vi "ESC Run VI Named.vi"(3 "Mode":T5=enum."Run VI", 5 "Traverse line In":T2={"Start X"=0.0, "Start Y"=0.0, "Start Z"=0.0, "End X"=0.0, "End Y"=0.0, "End Z"=0.0, "nPoints"=0, "Spacing"=enum."Linear", "Filename"=path "", "Tunnel Speed"=0.0, "Averaging time (mins)"=0.0, "Extra Commands"="", "Carrier_1 Q (l/min)"=0.0, "Carrier_2 Q (l/min)"=0.0, "Trace Gas Concentration (%)"=0.0, "Specific Arguments"="Source_Live_Control.vi; 1", "Comments"="", "Row No"=0, "Row Type Selector"=enum."Move Traverse Only", "EstCompl"="", "Row Duration (mins)"=0.0, "nValidPoints"=0, "Meas Setup File"=""} {"Carrier_2 Q (l/min)" format="%#.2f"; "Row Duration (mins)" format="%#.1f"; "Row No" min=0; "Trace Gas Concentration (%)" min=0.0 format="%#_4f"; "Carrier_1 Q (l/min)" format="%#.4f"; "Start X" format="%#.2f"; "Start Y" format="%#.2f"; "Start Z" format="%#.2f"; "End X" format="%#.2f"; "End Y" format="%#.2f"; "End Z" format="%#.2f"; "Tunnel Speed" format="%#.2f"; "Averaging time (mins)" min=0.0 format="%#.2f"}) -> (0 "Error Message":string, 1 "Status":T1, 2 "Traverse line Out":T2={"Start X"=0.0, "Start Y"=0.0, "Start Z"=0.0, "End X"=0.0, "End Y"=0.0, "End Z"=0.0, "nPoints"=0, "Spacing"=enum."Linear", "Filename"=path "", "Tunnel Speed"=0.0, "Averaging time (mins)"=0.0, "Extra Commands"="", "Carrier_1 Q (l/min)"=0.0, "Carrier_2 Q (l/min)"=0.0, "Trace Gas Concentration (%)"=0.0, "Specific Arguments"="Source_Live_Control.vi; 1", "Comments"="", "Row No"=0, "Row Type Selector"=enum."Move Traverse Only", "EstCompl"="", "Row Duration (mins)"=0.0, "nValidPoints"=0, "Meas Setup File"=""} {"Carrier_2 Q (l/min)" format="%#.2f"; "Row Duration (mins)" format="%#.1f"; "Row No" min=0; "Trace Gas Concentration (%)" min=0.0 format="%#_4f"; "Carrier_1 Q (l/min)" format="%#.4f"; "Start X" format="%#.2f"; "Start Y" format="%#.2f"; "Start Z" format="%#.2f"; "End X" format="%#.2f"; "End Y" format="%#.2f"; "End Z" format="%#.2f"; "Tunnel Speed" format="%#.2f"; "Averaging time (mins)" min=0.0 format="%#.2f"})   [LabVIEW 2022 SP3]
uses:
  Gen Trav/Traverse_cluster.ctl
  Gen Trav/Spacing.ctl
  Controls/Multi_run_mode.ctl
  Controls/User_Specific_mode.ctl
  Gen Trav/Multi_Run_Status.ctl
panel:
  out "Desired RPM":dbl
  # "X           Y          Z"
  # "Start"
  # "End"
  # "X           Y          Z"
  # "Start"
  # "End"
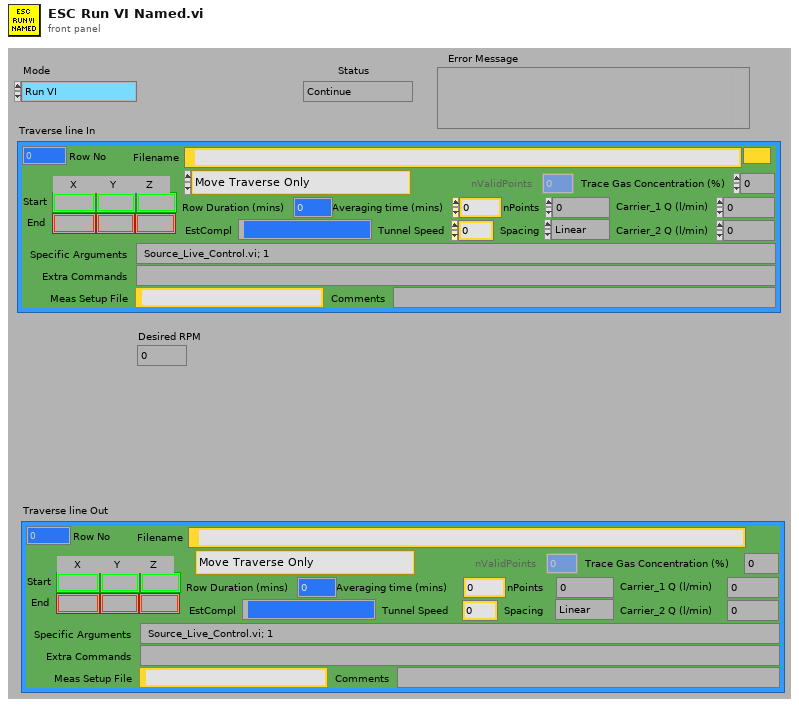
[diagram p1: front panel]
types:
  T1 = typedef "Multi_Run_Status.ctl" = enum16{"Continue", "Continue with Error", "Jump to Next Point", "Jump to Next Row", "Jump To Fall Back", "Terminate Run"}
  T2 = typedef "Traverse_cluster.ctl" = cluster{"Start X":sgl, "Start Y":sgl, "Start Z":sgl, "End X":sgl, "End Y":sgl, "End Z":sgl, "nPoints":i32, "Spacing":T3, "Filename":path, "Tunnel Speed":dbl, "Averaging time (mins)":dbl, "Extra Commands":string, "Carrier_1 Q (l/min)":dbl, "Carrier_2 Q (l/min)":dbl, "Trace Gas Concentration (%)":dbl, "Specific Arguments":string, "Comments":string, "Row No":i32, "Row Type Selector":T4, "EstCompl":string, "Row Duration (mins)":dbl, "nValidPoints":i32, "Meas Setup File":string}
  T3 = typedef "Spacing.ctl" = enum16{"Linear", "Log", "Gauss", "Specified", "N/A"}
  T4 = typedef "Multi_run_mode.ctl" = enum16{"Move Traverse Only", "Set Tunnel Speed Only", "Set Source Only", "Set Measurement Conditions", "Single Measurement", "Vertical Profile", "Lateral Profile", "Longitudinal Profile", "Multi-Axis Profile", "Explore Volume", "Auto Calibrate", "Meas Fast FID Bkgnd", "Check Beam Power", "Scanning Valve Measurement", "Run VI Named:", "Set ADAM Ch", "Wait (minutes)", "Send Message", "Synchronize With:", "Fall Back to this Row", "Turn Off Row Repeating", "Traverse 3D Volume", "Blank Row", "Jump to Fall Back Row"}
  T5 = typedef "User_Specific_mode.ctl" = enum16{"Check VI only", "Run VI"}
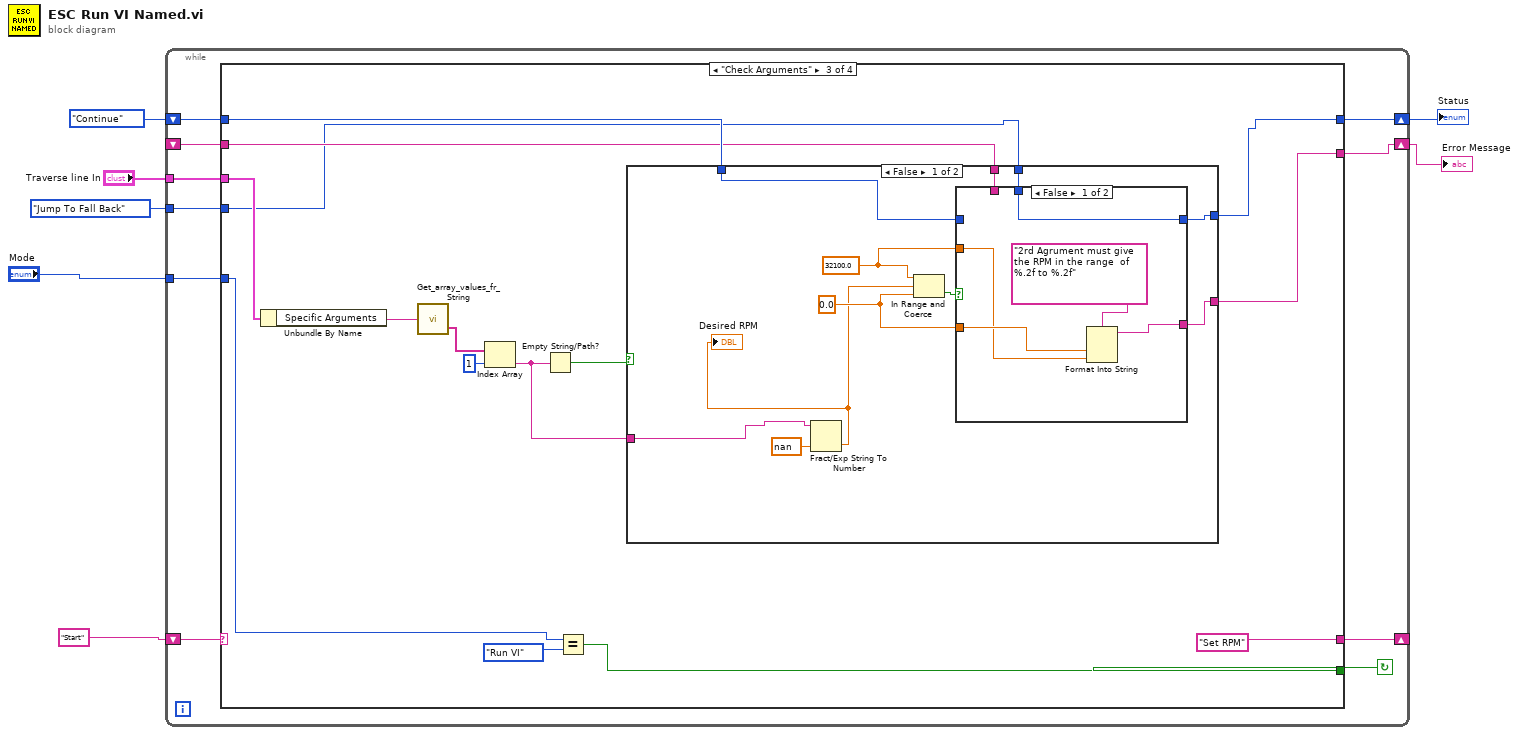
[diagram p0: block diagram]
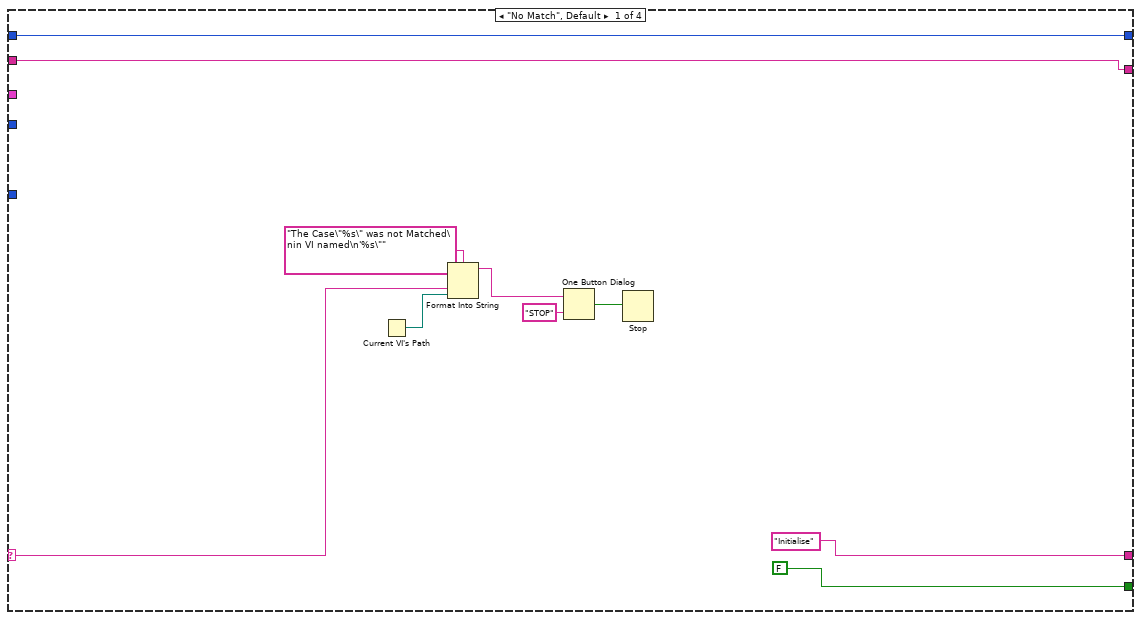
[diagram p2: hidden frame]
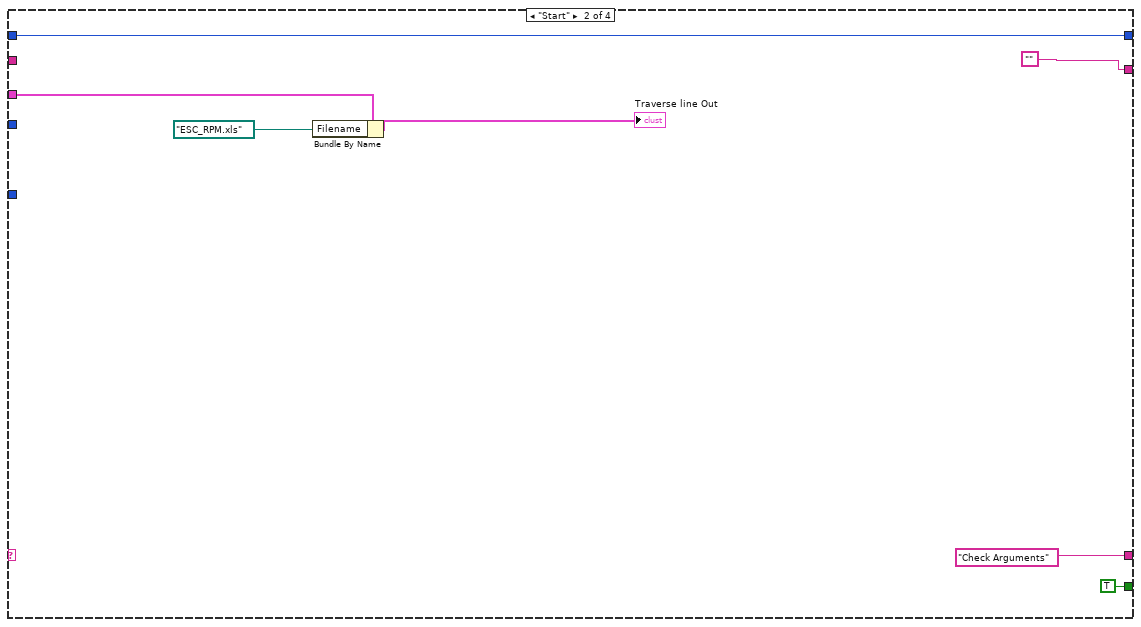
[diagram p3: hidden frame]
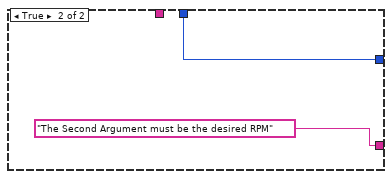
[diagram p5: hidden frame]
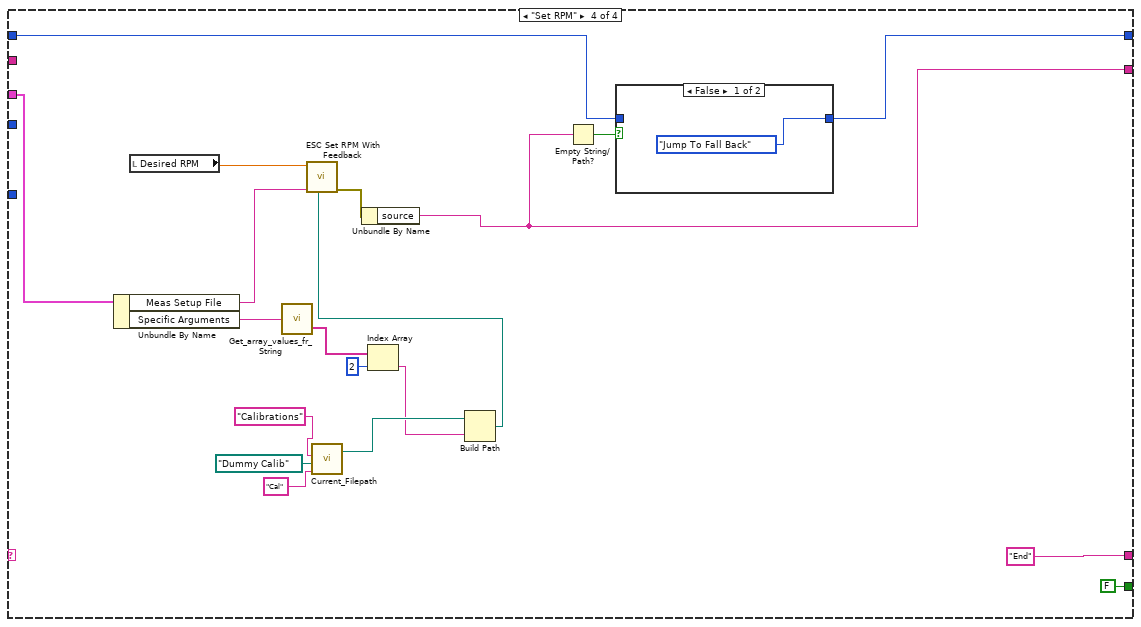
[diagram p6: hidden frame]
diagram:
  n1 = while {
    shift-left: "Start" -> [w15]
    shift-right: [w16] -> _
    tunnel: "Mode" -> [w14]
    shift-right: [w13] -> w5
    shift-left: Multi_Run_Status."Continue" ("Status") -> [w11]
    shift-right: [w12] -> w4
    shift-left: _ -> [w10]
    tunnel: "Traverse line In" -> [w9]
    tunnel: Multi_Run_Status."Jump To Fall Back" ("Status") -> [w8]
    stop <- w17 continue-if-true
    n2 = case shown="\"Check Arguments\"" w15 {
      selector: w15 -> [w20 _ _ _]
      tunnel: [FALSE TRUE ("Power Control?") w39 FALSE ("Power Control?")] -> w17
      tunnel: ["Initialise" "Check Arguments" "Set RPM" "End"] -> w16
      tunnel: w14 -> [_ _ w40 _]
      tunnel: [w19 w33 w45 w84] -> w13
      tunnel: [w18 "" w46 w79] -> w12
      tunnel: w11 -> [w19 w33 w43 w83]
      tunnel: w10 -> [w18 _ w42 _]
      tunnel: w9 -> [_ w30 w47 w82]
      tunnel: w8 -> [_ _ w38 _]
      frame "No Match", Default {
        n3 = Current VI's Path() -> (path=w22:path)
        n4 = Format Into String(format string="The Case\"%s\" was not Matched\nin VI named\n'%s\"" ("Format String"), w20, w22) -> (resulting string=w25:string)  [unwired: 2 in, 1 out]
        n5 = One Button Dialog(message=w25, button name ("OK")="STOP") -> (true=w23:bool)
        n6 = Stop(stop? (T)=w23) -> ()
      }
      frame "Start" {
        n7 = Bundle By Name(cluster=w30, "Filename"=path "ESC_RPM.xls" ("Results Filename")) -> (→"Traverse line Out":T2)
      }
      frame "Check Arguments" {
        n8 = Unbundle By Name(w47) -> ("Specific Arguments"=w48:string)
        n9 = call "Get_array_values_fr_String.vi"("String Value"=w48) -> ("String array"=w44:string[])  [unwired: 1 out]
        n10 = Index Array(array=w44, index=1) -> (element=w35:string)
        n11 = Empty String/Path?(string/path=w35) -> (empty?=w37:bool)
        n12 = Equal?(x=w40, y=User_Specific_mode."Run VI" ("Mode")) -> (x = y?=w39:bool)
        n13 = case shown="False" w37 {
          tunnel: [w56 "The Second Argument must be the desired RPM" ("format string")] -> w46
          tunnel: [w55 w69] -> w45
          tunnel: w43 -> [w54 _]
          tunnel: w42 -> [w53 _]
          tunnel: w38 -> [w51 w69]
          tunnel: w35 -> [w50 _]
          frame False {
            w57 = 32100.0
            w58 = 0.0
            n14 = Fract/Exp String To Number(string=w50, default (0 dbl)=nan ("default (0 DBL)")) -> (number=w52:dbl)  [unwired: 2 in, 1 out]
            "Desired RPM" <- w52
            n15 = In Range and Coerce(upper limit=w57, x=w52, lower limit=w58) -> (In Range?=w59:bool)  [unwired: 1 out]
            n16 = case shown="False" w59 {
              tunnel: w58 -> [w64 _]
              tunnel: w57 -> [w63 _]
              tunnel: [w62 w66] -> w56
              tunnel: [w61 w67] -> w55
              tunnel: w54 -> [_ w67]
              tunnel: w53 -> [_ w66]
              tunnel: w51 -> [w61 _]
              frame False {
                n17 = Format Into String(format string="2rd Agrument must give the RPM in the range  of %.2f to %.2f", w64, w63) -> (resulting string=w62:string)  [unwired: 2 in, 1 out]
              }
              frame True {
              }
            }
          }
          frame True {
          }
        }
      }
      frame "Set RPM" {
        n18 = Unbundle By Name(w82) -> ("Meas Setup File"=w81:string, "Specific Arguments"=w73:string)
        n19 = local read "Desired RPM"() -> (w86:dbl)
        n20 = call "Get_array_values_fr_String.vi"("String Value"=w73) -> ("String array"=w74:string[])  [unwired: 1 out]
        n21 = call "Current_Filepath.vi"("Short_Name"="Cal" ("Data Type"), "Filename in"=path "Dummy Calib", "Data Type"="Calibrations") -> ("Directory"=w72:path)  [unwired: 1 in, 1 out]
        n22 = Index Array(array=w74, index=2) -> (element=w71:string)
        n23 = Build Path(base path=w72, name or relative path=w71) -> (appended path=w70:path)
        n24 = call "ESC Set RPM With Feedback.vi"("Calib File"=w70, "Meas Setup filename"=w81, "Desired RPM"=w86) -> ("Error Out"=w80:errorcluster)  [unwired: 6 in, 2 out]
        n25 = Unbundle By Name(w80) -> ("source"=w79:string)
        n26 = Empty String/Path?(string/path=w79) -> (empty?=w85:bool)
        n27 = case shown="False" w85 {
          tunnel: [Multi_Run_Status."Jump To Fall Back" ("Status") w90] -> w84
          tunnel: w83 -> [_ w90]
          frame False {
          }
          frame True {
          }
        }
      }
    }
  }
  "Error Message" <- w4
  "Status" <- w5
